vi "Exit For Loop.vi"(0 "Diagram in":refnum<vi>, 1 "Conditional Terminals":refnum<vi>[](array[refnum]), 2 "Loop Terminal Types":T1[](array[typedef]), 5 "Outputs":refnum<vi>[](array[refnum]), 7 "Shift Registers":refnum<vi>[](array[refnum]), 9 "Stop Condition":refnum<vi>, 11 "error in (no error)":errorcluster) -> (4 "Diagram out":refnum<vi>, 6 "Outputs":refnum<vi>[](array[refnum]), 8 "Shift Registers":refnum<vi>[](array[refnum]), 15 "error out":errorcluster)   [LabVIEW 2015, in "Scripting.lvlib"]
doc: "Exits the For Loop that owns <B>Diagram in</B>, supplying the structure's owning diagram at <B>Diagram out</B>.\n\n<B>Stop Condition</B> is optionally the terminal to wire to the conditional terminal of the For Loop.\n\n<B>Conditional Terminals</B> is optionally an array of terminals to wire to the conditional terminal of the For Loop's output tunnels.\n\n<B>Loop Terminal Types</B> is optionally and array of terminal types of the For Loop's output tunnels."
uses:
  Scripting.lvlib
  Loop Terminal Type.ctl
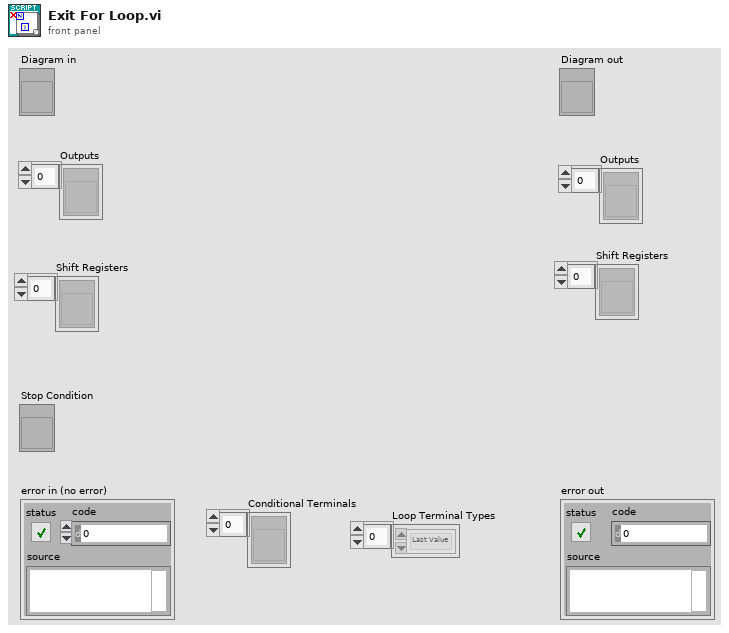
[diagram p1: front panel]
types:
  T1 = typedef "Scripting.lvlib/Loop Terminal Type.ctl" = enum16{"Last Value", "Indexing", "Concatenating"}
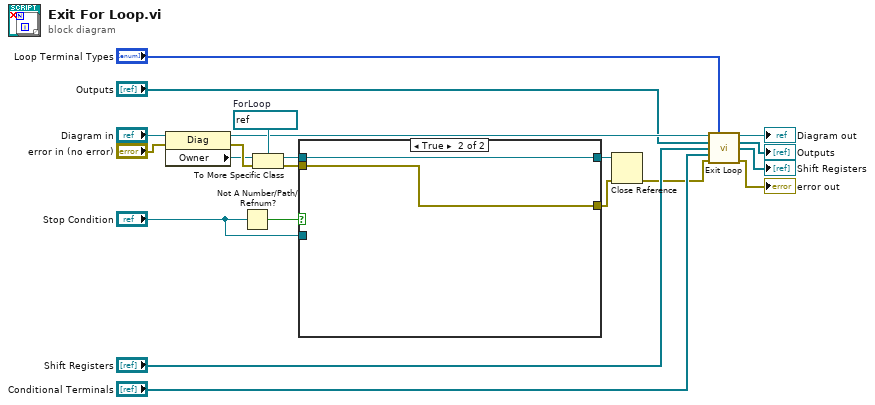
[diagram p0: block diagram]
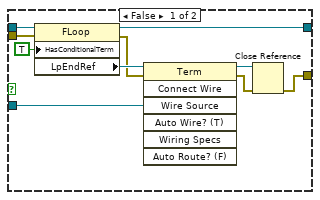
[diagram p2: hidden frame]
diagram:
  w20 = refnum<vi> refnum  # ForLoop
  n1 = property class="Diag"(reference="Diagram in", error in="error in (no error)") -> (reference out=w16:refnum<vi>, error out=w21:errorcluster, "Owner"=w19:refnum<vi>)
  n2 = Not A Number/Path/Refnum?(number/path/refnum="Stop Condition") -> (NaN/Path/Refnum?=w13:bool)
  n3 = To More Specific Class(target class=w20, reference=w19, error in=w21) -> (specific class reference=w9:refnum<vi>, error out=w8:errorcluster)
  n4 = case shown="True" w13 {
    tunnel: "Stop Condition" -> [w31 _]
    tunnel: [w23 w33] -> w1
    tunnel: w9 -> [w29 w32]
    tunnel: w8 -> [w28 w33]
    tunnel: [w24 w32] -> w3
    frame False {
      n5 = property class="FLoop"(reference=w29, error in=w28, "HasConditionalTerm"=TRUE ("Has Conditional Terminal?")) -> (reference out=w24:refnum<vi>, error out=w25:errorcluster, "LpEndRef"=w26:refnum<vi>)
      n6 = invoke class="Term" method="Connect Wire"(reference=w26, error in=w25, "Wire Source"=w31) -> (reference out=w22:refnum<vi>, error out=w30:errorcluster)  [unwired: 4 in, 5 out]
      n7 = Close Reference(reference=w22, error in (no error)=w30) -> (error out=w23:errorcluster)
    }
    frame True {
    }
  }
  n8 = Close Reference(reference=w3, error in (no error)=w1) -> (error out=w2:errorcluster)
  n9 = call "Exit Loop.vi"("Diagram in"=w16, "Loop Terminal Types"="Loop Terminal Types", "Outputs"="Outputs", "Shift Registers"="Shift Registers", "Conditional Terminals"="Conditional Terminals", "error in (no error)"=w2) -> ("Diagram out"=→"Diagram out":refnum<vi>, "Outputs"=→"Outputs":refnum<vi>[], "Shift Registers"=→"Shift Registers":refnum<vi>[], "error out"=→"error out":errorcluster)  [unwired: 6 in]
